vi "Create MetaData Channel - Single Channel - Enumerated List.vi"(8 "error in (no error)":errorcluster, 9 "settings":T2, 10 "channel name":string, 11 "command refnum in":T1=18446744073709551615 format="%.0x") -> (0 "error out":errorcluster, 2 "channel refnum":T1=18446744073709551615 format="%.0x", 3 "command refnum out":T1=18446744073709551615 format="%.0x")   [LabVIEW 2019, in "Instrument Addon Scripting API.lvlib"]
doc: "Creates a new MetaData Channel under the specified command."
uses:
  Instrument Addon Scripting API.lvlib
  <vilib>/NI VeriStand/Custom Device API/Custom Device Item Ref.ctl
  TypeDefs/Single Channel Enumerated List Settings.ctl
  Addon/Addon Shared/Types/MetaData Parameters.ctl
  Addon/Addon Shared/Types/Protocol Data Type.ctl
  Addon/Addon Shared/Types/Metadata Channel Type.ctl
  Addon/Addon Shared/Types/Type Cast Type.ctl
  Addon/Addon Shared/Types/Endian.ctl
  TypeDefs/Channel Properties.ctl
  Addon/Addon Shared/Instrument Addon Shared.lvlib
  <vilib>/NI VeriStand/Custom Device API/Custom Device API.lvlib
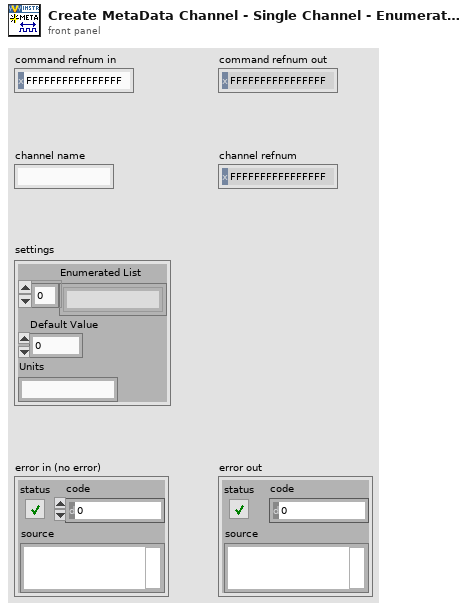
[diagram p1: front panel]
types:
  T1 = typedef "Custom Device API.lvlib/Custom Device Item Ref.ctl" = u64
  T2 = typedef "Instrument Addon Scripting API.lvlib/Single Channel Enumerated List Settings.ctl" = cluster{"Enumerated List":string[], "Default Value":dbl, "Units":string}
  T3 = typedef "Instrument Addon Scripting API.lvlib/Channel Properties.ctl" = cluster{"Default Value":dbl, "Units":string}
  T4 = typedef "Instrument Addon Shared.lvlib/Metadata Channel Type.ctl" = enum16{"Enumerated List", "Format", "Type Cast"}
  T5 = typedef "Instrument Addon Shared.lvlib/Protocol Data Type.ctl" = enum16{"Single Channel", "Array"}
  T6 = typedef "Instrument Addon Shared.lvlib/MetaData Parameters.ctl" = cluster{"Data Type":T5, "Channel Type":T4, "List":string[], "Format String":string, "Type":T7, "Delimiter":string, "Endian":T8}
  T7 = typedef "Instrument Addon Shared.lvlib/Type Cast Type.ctl" = enum16{"DBL", "SGL", "U64", "U32", "U16", "U8", "I64", "I32", "I16", "I8"}
  T8 = typedef "Instrument Addon Shared.lvlib/Endian.ctl" = enum16{"Native", "Little", "Big"}
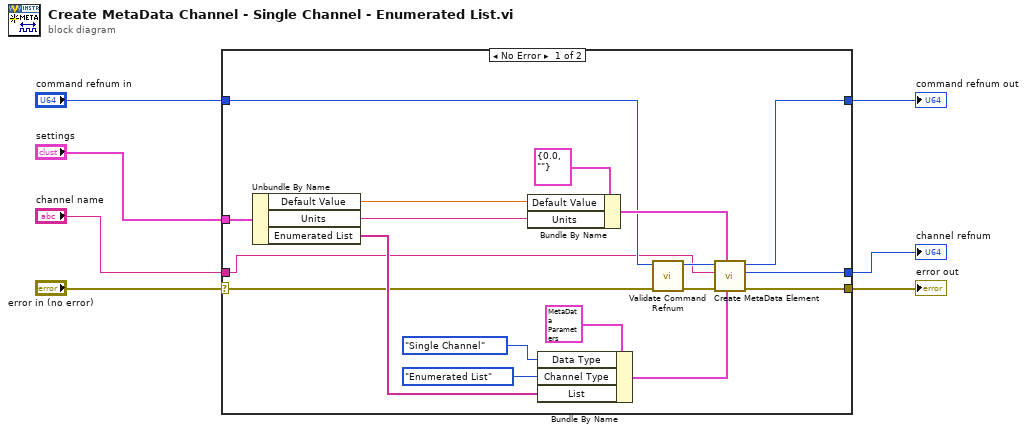
[diagram p0: block diagram]
diagram:
  n1 = case shown="No Error" "error in (no error)" {
    selector: "error in (no error)" -> [w9 w26]
    tunnel: [w25 w26] -> w7
    tunnel: "settings" -> [w24 _]
    tunnel: "command refnum in" -> [w12 w27]
    tunnel: [w14 _] -> w4
    tunnel: [w13 w27] -> w3
    tunnel: "channel name" -> [w8 _]
    frame No Error {
      n2 = Unbundle By Name(w24) -> ("Default Value"=w18:dbl, "Units"=w17:string, "Enumerated List"=w20:string[])
      n3 = Bundle By Name(cluster=T3 {"Default Value"=0.0, "Units"=""}, "Default Value"=w18, "Units"=w17) -> (w15:T3)
      n4 = Bundle By Name(cluster=T6 {"Data Type"=enum."Single Channel", "Channel Type"=enum."Format", "List"=[], "Format String"="%.3g", "Type"=enum."SGL", "Delimiter"="", "Endian"=enum."Native"} ("MetaData Parameters"), "Data Type"=Protocol_Data_Type."Single Channel", "Channel Type"=Metadata_Channel_Type."Enumerated List", "List"=w20) -> (w19:T6)
      n5 = call "Validate Command Refnum.vi"("error in (no error)"=w9, "command refnum in"=w12) -> ("error out"=w10:errorcluster, "command refnum out"=w11:T1)  [unwired: 8 in]
      n6 = call "Create MetaData Element.vi"("MetaData Parameters"=w19, "Channel Properties"=w15, "error in (no error)"=w10, "Name"=w8, "Refnum In"=w11) -> ("error out"=w25:errorcluster, "Channel Refnum"=w14:T1, "Refnum Out"=w13:T1)  [unwired: 4 in]
    }
    frame Error {
    }
  }
  "command refnum out" <- w3
  "error out" <- w7
  "channel refnum" <- w4
